vi "ConvertTextBasedCodeToLabVIEW.vi"() -> ()   [LabVIEW 2012]
uses:
  <resource>/Framework/Providers/Open_GDS/ClassProviders/Common/String/GDSString_ClassDescriptionType.ctl
  <resource>/Framework/Providers/Open_GDS/ClassProviders/Common/String/GDSString_AccessScopeModifierType.ctl
  <resource>/Framework/Providers/Open_GDS/ClassProviders/Common/String/GDSString_ModifierType.ctl
  <resource>/Framework/Providers/Open_GDS/ClassProviders/Common/String/GDSString_MethodDescriptionType.ctl
  <resource>/Framework/Providers/Open_GDS/ClassProviders/Common/String/GDSString_ClassParentType.ctl
  <resource>/Framework/Providers/Open_GDS/ClassProviders/Common/String/GDSString_ClassType.ctl
  <resource>/Framework/Providers/Open_GDS/ClassProviders/Common/String/GDSString_ClassOwnerType.ctl
  <resource>/Framework/Providers/Open_GDS/ClassProviders/Common/CommonVIs/CommonVIs_AttributeType.ctl
  <resource>/Framework/Providers/Open_GDS/ClassProviders/Common/CommonVIs/CommonVIs_AttributeDataType.ctl
  <resource>/Framework/Providers/Open_GDS/ClassProviders/Common/CommonVIs/CommonVIs_EnumType.ctl
  <resource>/Framework/Providers/Open_GDS/ClassProviders/Common/CommonVIs/CommonVIs_StructType.ctl
  <vilib>/Utility/miscctls.llb/LVPointTypeDef.ctl
  <vilib>/Platform/browser.llb/Open URL in Default Browser (path).vi
panel:
  out "Array":T1[](array[typedef])
  out "Classes":T4[](array[typedef])
  out "Tab":T12(tab)
  in  "RemoveSelectedFiles":bool
  in  "ClearList":bool
  in  "FileList":i32[](listbox) caption="File List"
  in  "CopyfromClipboard":bool
  in  "Code":string caption="Java or C# Code"
  in  "Path":path caption="Java or C# File or top level folder"
  out "FileListText":bool
  in  "Missing":i32(listbox) caption="Missing Classes and types"
  in  "ViewClassOverView":bool
  in  "ClassType":T13(ring) caption="Class Type"
  in  "TopFolder":path caption="Top Folder for all classes"
  in  "Previous":bool
  in  "Cancel":bool
  in  "Next":bool
  out "error IO":errorcluster
  # "There are some missing classes/types that could not be found.\nDo you want to contine?\nYou can go back and add some more files that might contain the missing types."
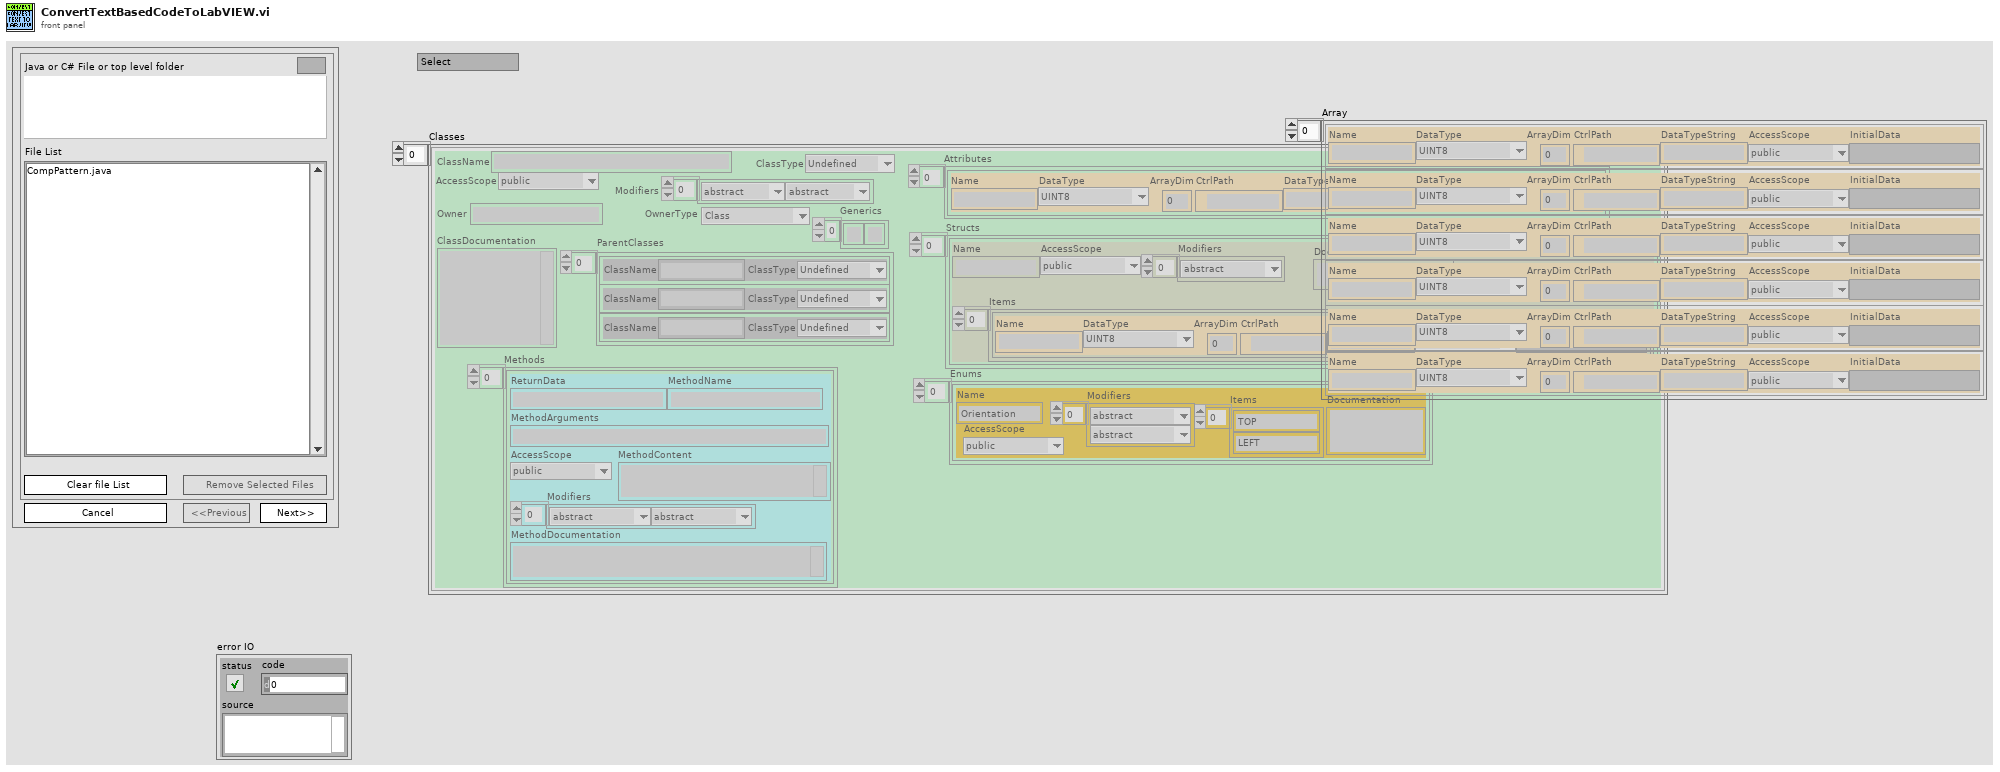
[diagram p1: front panel]
types:
  T1 = typedef "CommonVIs_AttributeType.ctl" = cluster{"Name":string, "DataType":T2, "ArrayDim":i32, "CtrlPath":path, "DataTypeString":string, "AccessScope":T3, "InitialData":variant}
  T2 = typedef "CommonVIs_AttributeDataType.ctl" = enum16{"UINT8", "INT8", "UINT16", "INT16", "UINT32", "INT32", "UINT64", "INT64", "SGL", "DBL", "EXT", "CSG", "CDB", "CXT", "TimeStamp", "STRING", "PATH", "BOOL", "ENUM", "RefNum", "VIRefNum", "LabVIEW Class", "Cluster", "Variant", "TypeDef", "Waveform", "LabVIEW Object", "Other"}
  T3 = typedef "GDSString_AccessScopeModifierType.ctl" = enum16{"public", "private", "protected", "internal"}
  T4 = typedef "GDSString_ClassDescriptionType.ctl" = cluster{"ClassName":string, "AccessScope":T3, "Modifiers":T5[], "ClassDocumentation":string, "Methods":T6[], "ParentClasses":T7[], "ClassType":T8, "Owner":string, "OwnerType":T9, "Generics":string[], "Attributes":T1[], "Enums":T10[], "Structs":T11[]}
  T5 = typedef "GDSString_ModifierType.ctl" = enum16{"abstract", "static", "final", "synchronized", "strictfp", "async", "const", "event", "extern", "new", "override", "partial", "readonly", "sealed", "unsafe", "virtual", "volatile"}
  T6 = typedef "GDSString_MethodDescriptionType.ctl" = cluster{"ReturnData":string, "MethodName":string, "MethodArguments":string, "AccessScope":T3, "Modifiers":T5[], "MethodDocumentation":string, "MethodContent":string}
  T7 = typedef "GDSString_ClassParentType.ctl" = cluster{"ClassName":string, "ClassType":T8}
  T8 = typedef "GDSString_ClassType.ctl" = enum16{"Undefined", "Class", "Interface"}
  T9 = typedef "GDSString_ClassOwnerType.ctl" = enum16{"NoOwner", "Class", "Package/NameSpace"}
  T10 = typedef "CommonVIs_EnumType.ctl" = cluster{"Name":string, "AccessScope":T3, "Modifiers":T5[], "Items":string[], "Documentation":string}
  T11 = typedef "CommonVIs_StructType.ctl" = cluster{"Name":string, "AccessScope":T3, "Modifiers":T5[], "Items":T1[], "Documentation":string}
  T12 = enum32{"Select", "Analysing", "Missing", "Overview"}
  T13 = enum16{"Native By Value LabVIEW Classes", "Reference Object DVR (GOOP4)", "Reference Object  (GOOP3)"}
  T14 = typedef "LVPointTypeDef.ctl" = cluster{"Horizontal":i16, "Vertical":i16}
  T15 = cluster{"Counter":i32, "Text":string, "Cancelled":bool, "Files":path[], "Classes":T4[]}
  T16 = enum8{"Enabled", "Disabled", "Disabled and Grayed Out"}
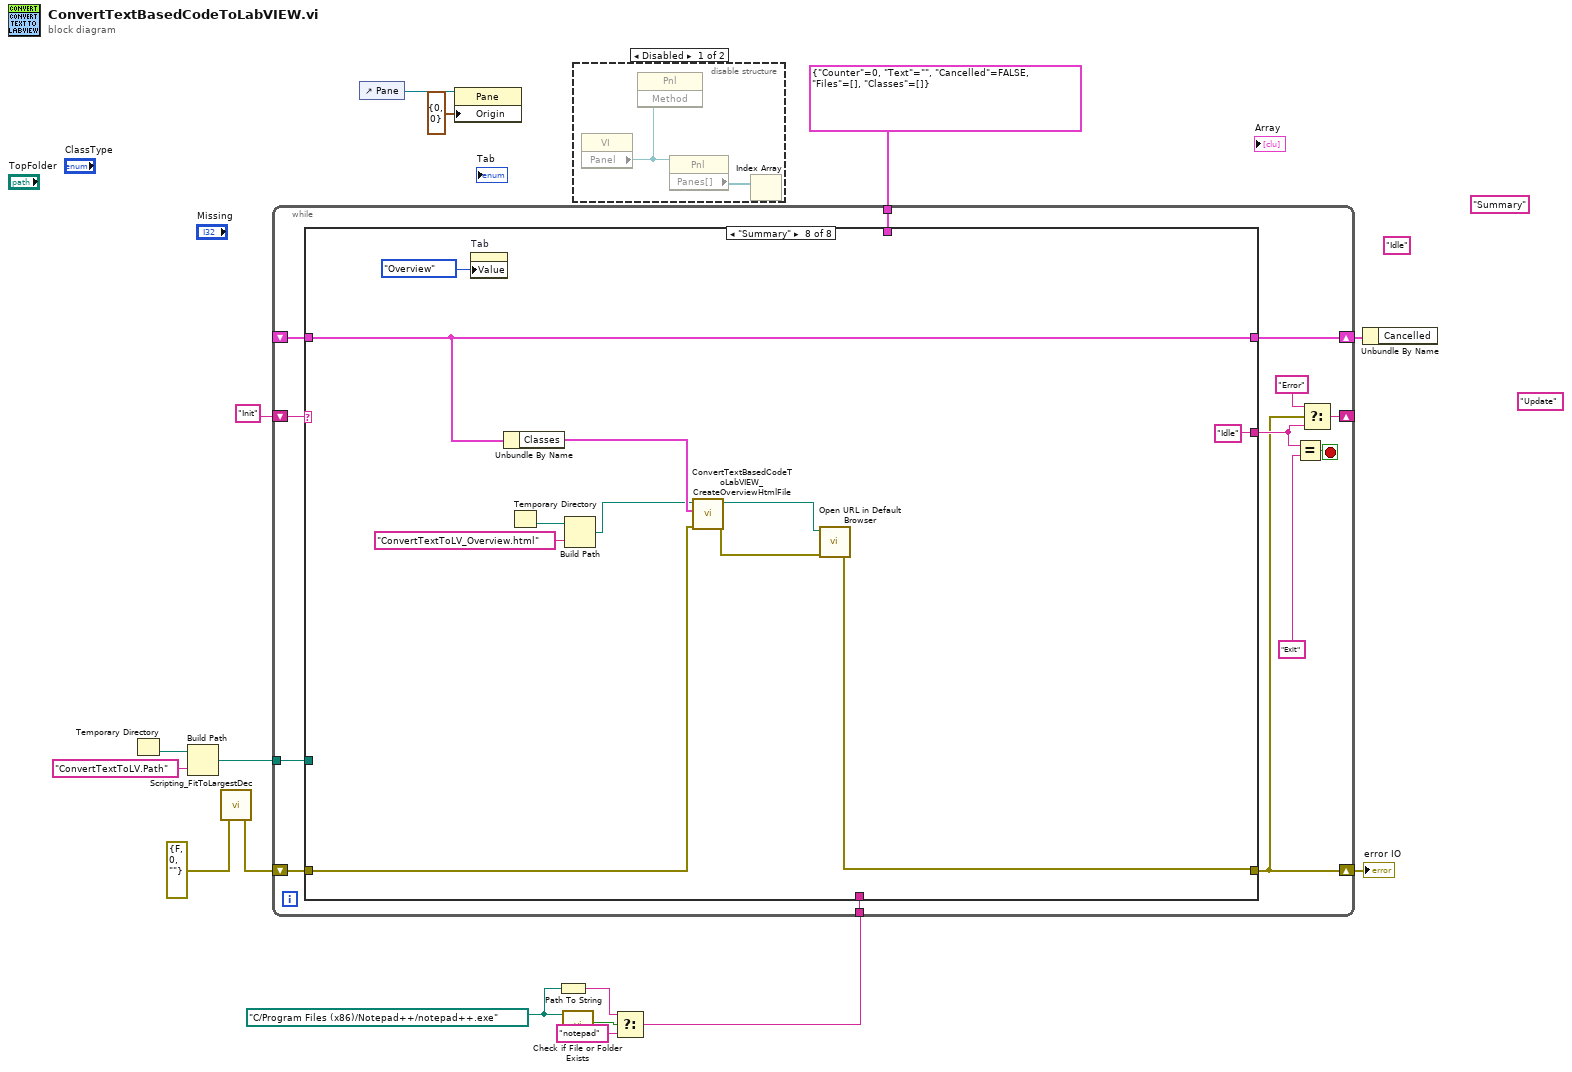
[diagram p0: block diagram]
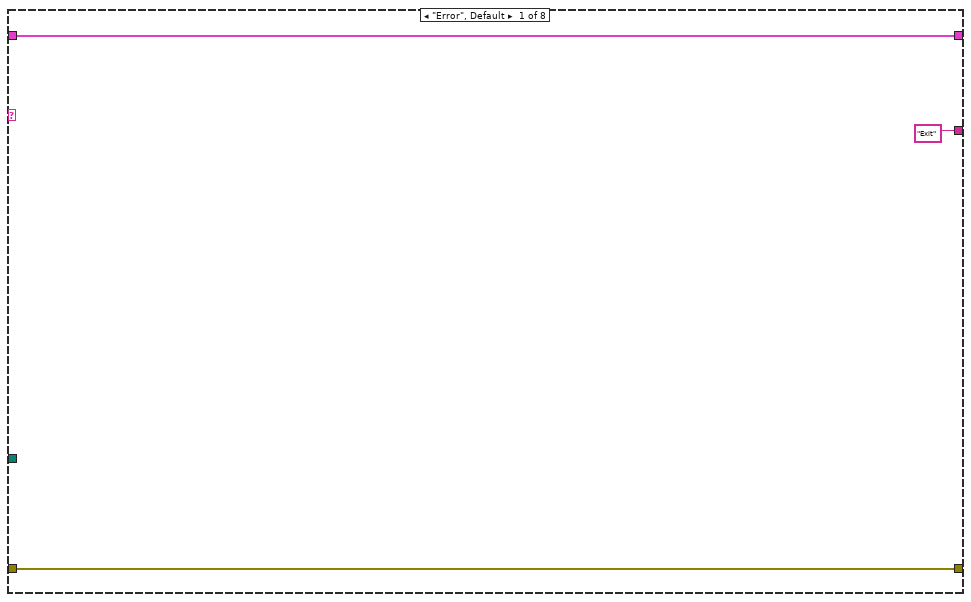
[diagram p3: hidden frame]
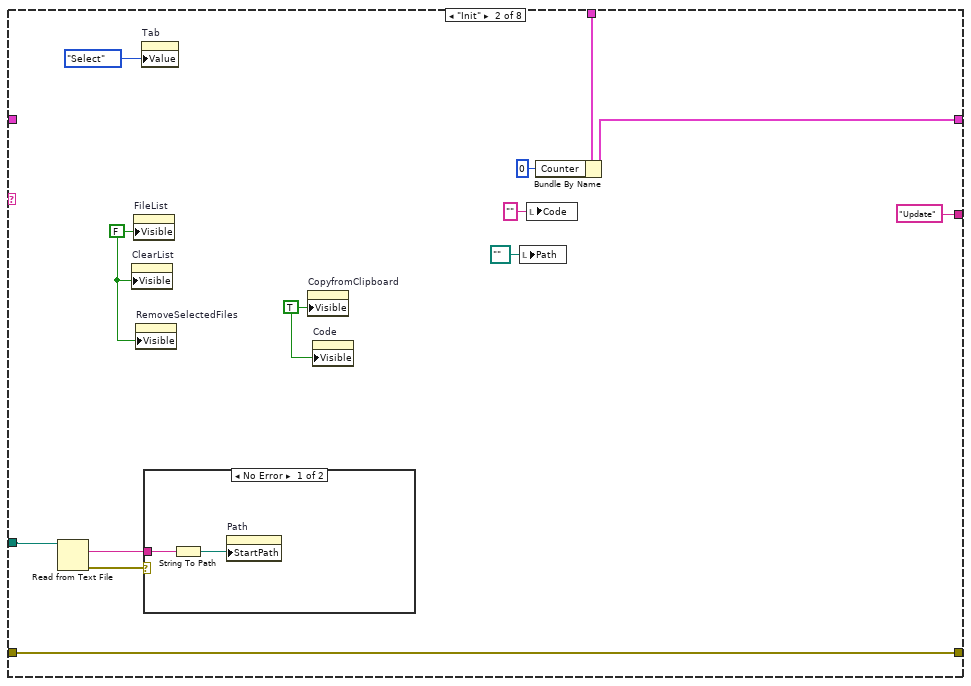
[diagram p4: hidden frame]
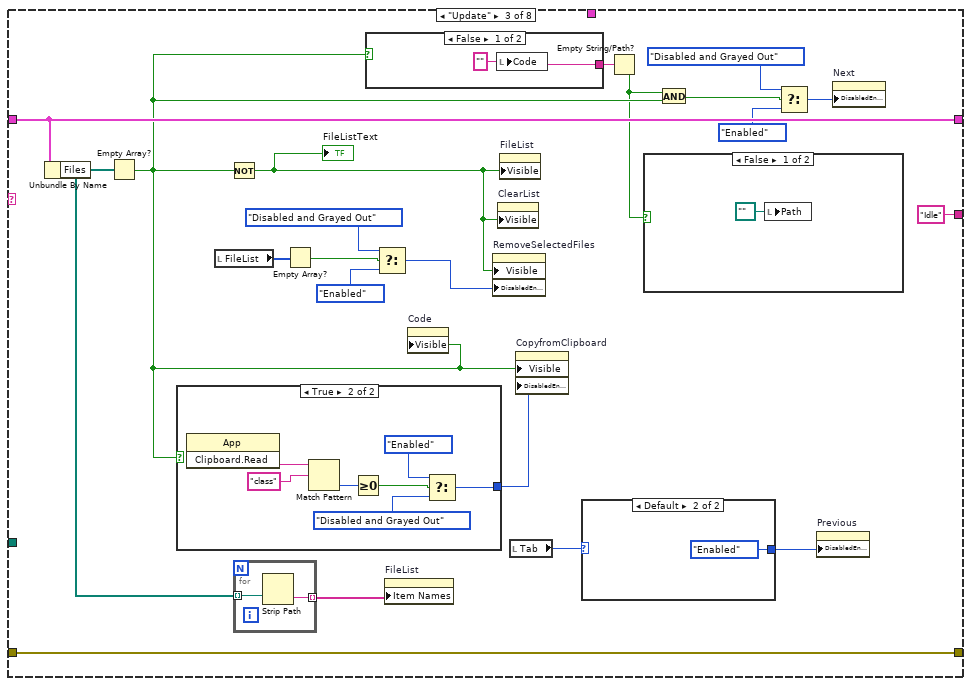
[diagram p6: hidden frame]
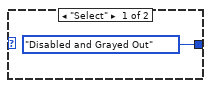
[diagram p7: hidden frame]
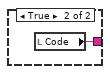
[diagram p9: hidden frame]
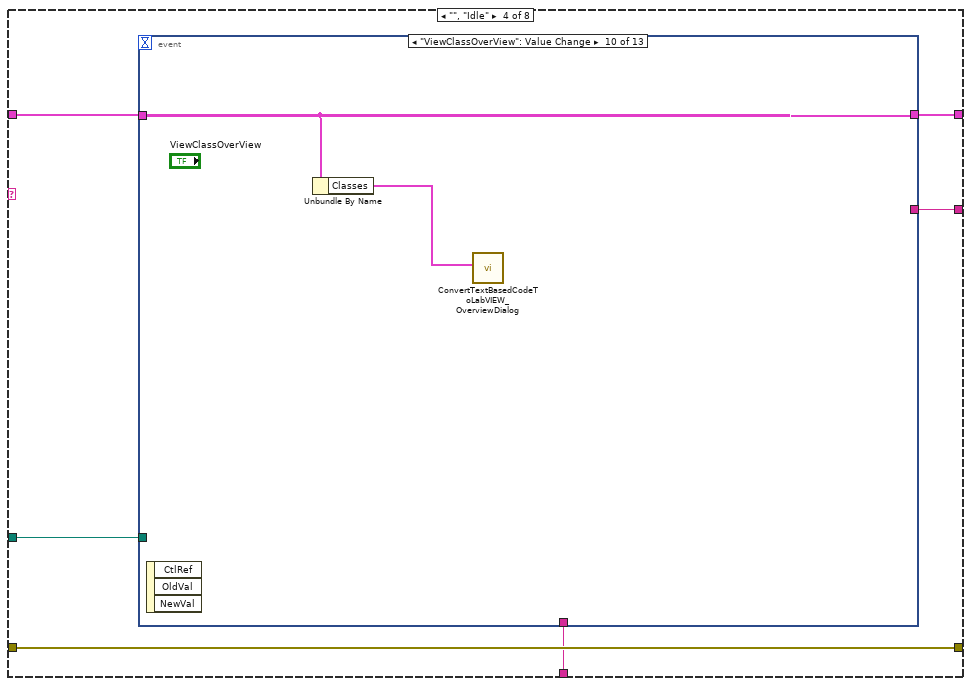
[diagram p11: hidden frame]
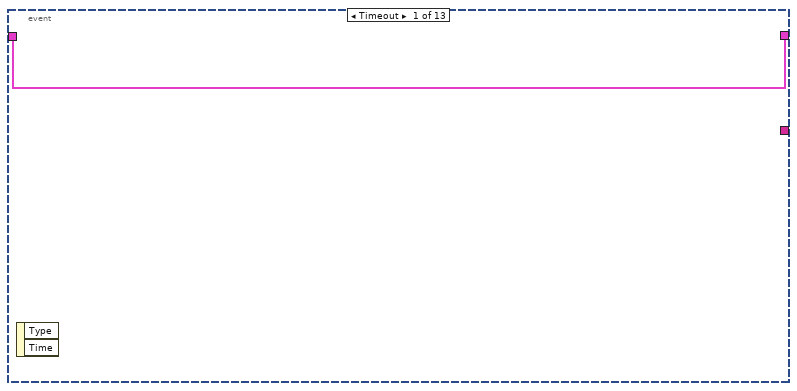
[diagram p12: hidden frame]
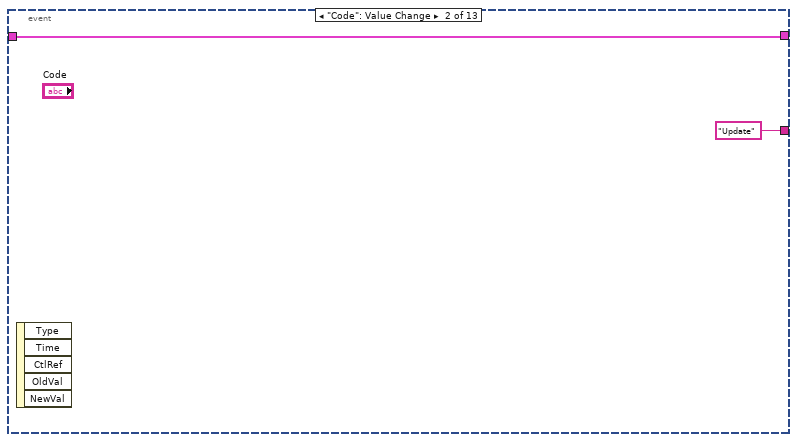
[diagram p13: hidden frame]
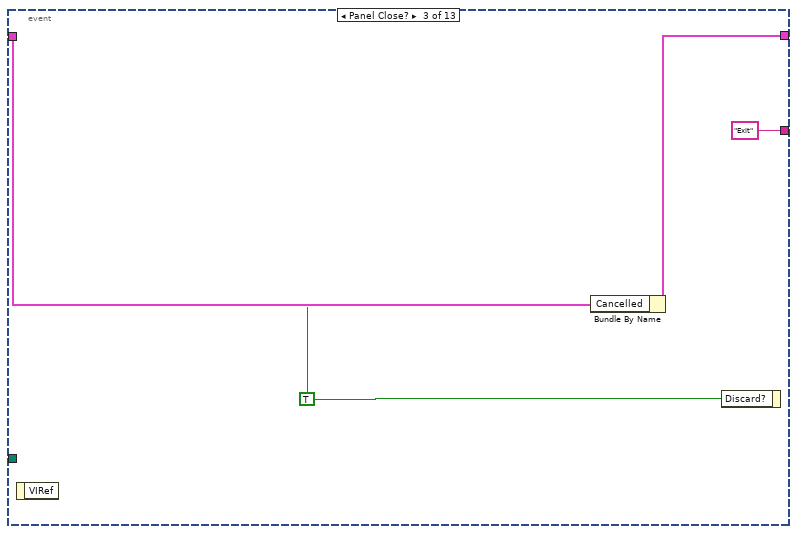
[diagram p14: hidden frame]
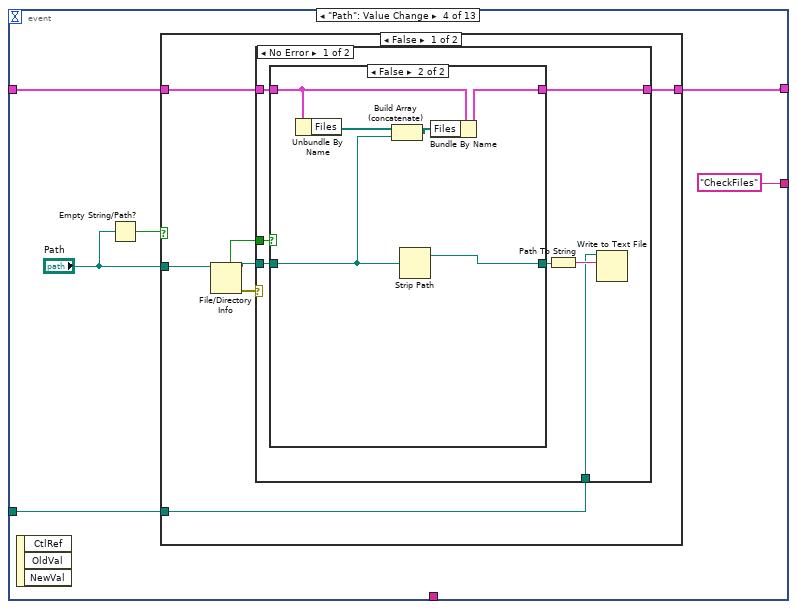
[diagram p15: hidden frame]
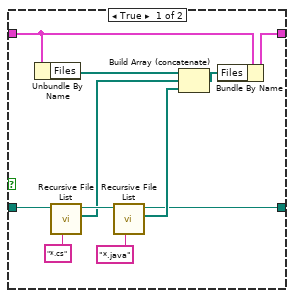
[diagram p16: hidden frame]
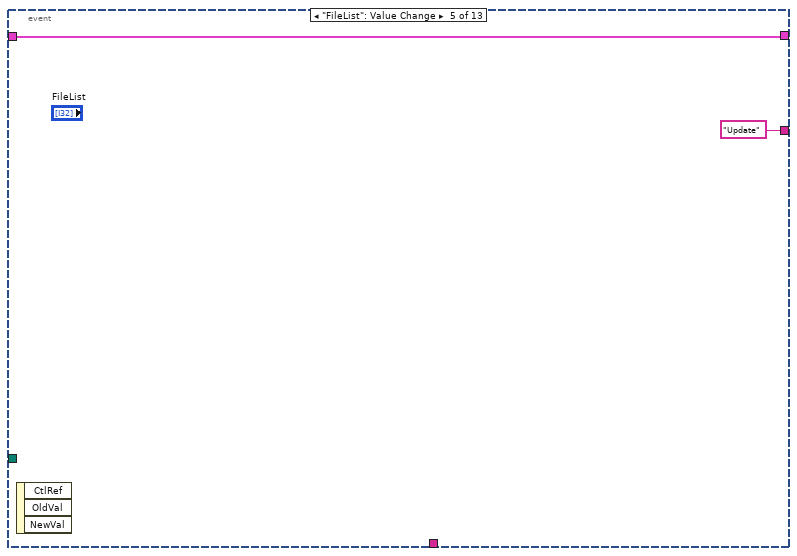
[diagram p19: hidden frame]
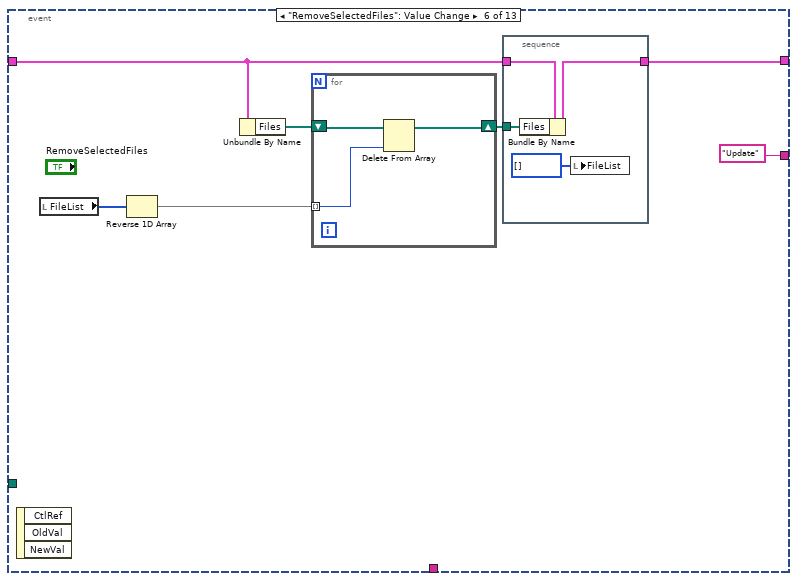
[diagram p20: hidden frame]
diagram:
  w4 = path "C:/Program Files (x86)/Notepad++/notepad++.exe"
  (unwired) "Update"
  (unwired) "Idle"
  (unwired) "Summary"
  n1 = Temporary Directory() -> (w9:path)
  n2 = Build Path(base path=w9, name or relative path="ConvertTextToLV.Path") -> (appended path=w8:path)
  n3 = call <resource>:"Scripting_FitToLargestDec.vi"("error in (no error)"=errorcluster {"status"=FALSE, "code"=0, "source"=""} ("error IO")) -> ("error out"=w6:errorcluster)  [unwired: 5 in, 1 out]
  n4 = control-ref of="Pane"() -> (w11:refnum<vi>)
  n5 = property class="Pane"(reference=w11, "Origin"=T14 {"Horizontal"=0, "Vertical"=0}) -> ()  [unwired: 1 in, 2 out]
  n6 = Path To String(path=w4) -> (string=w3:string)
  n7 = call <vilib>:"Check if File or Folder Exists.vi"("path"=w4) -> ("file or folder exists?"=w5:bool)  [unwired: 8 in, 2 out]
  n8 = disable-structure shown="Disabled" {
    frame Disabled {
      n9 = property class="VI"() -> ("Panel"=w18:refnum<vi>)  [unwired: 2 in, 2 out]
      n10 = invoke class="Pnl" method=#-1(reference=w18) -> ()  [unwired: 2 in, 3 out]
      n11 = property class="Pnl"(reference=w18) -> ("Panes[]"=w17:refnum<vi>[])  [unwired: 1 in, 2 out]
      n12 = Index Array(array=w17) -> ()  [unwired: 1 in, 1 out]
    }
    frame Enabled {
    }
  }
  n13 = Select(t=w3, s=w5, f="notepad") -> (s? t:f=w1:string)
  n14 = while {
    shift-right: [w24] -> w14
    shift-left: w6 -> [w31]
    shift-right: [w29] -> _
    shift-left: "Init" -> [w30]
    shift-right: [w23] -> w15
    shift-left: _ -> [w22]
    tunnel: T15 {"Counter"=0, "Text"="", "Cancelled"=FALSE, "Files"=[], "Classes"=[]} -> [w21]
    tunnel: w8 -> [w20]
    tunnel: w1 -> [w19]
    stop <- w28 stop-if-true
    n15 = case shown="\"Summary\"" w30 {
      tunnel: w31 -> [w34 w46 w68 w87 w215 w235 w307 w323]
      tunnel: [w34 w46 w68 w87 w214 w236 w307 w322] -> w24
      tunnel: ["Exit" "Update" "Idle" w88 w207 w237 "Update" "Idle"] -> w25
      tunnel: [w32 w45 w69 w89 w208 w246 w308 w328] -> w23
      tunnel: w22 -> [w32 _ w69 w90 w213 w246 w310 w328]
      tunnel: w21 -> [_ w43 _ _ _ _ _ _]
      tunnel: w20 -> [_ w38 _ w86 _ _ _ _]
      tunnel: w19 -> [_ _ _ w85 _ _ _ _]
      frame "Error", Default {
      }
      frame "Init" {
        w39 = TRUE ("Visible")
        w40 = FALSE ("Visible")
        n16 = Read from Text File(file (use dialog)=w38) -> (text=w36:string, error out=w37:errorcluster)  [unwired: 3 in, 2 out]
        n17 = property on="ClearList" class="Bool"("Visible"=w40) -> ()  [unwired: 2 in, 2 out]
        n18 = property on="FileList" class="LstBox (strict)"("Visible"=w40) -> ()  [unwired: 2 in, 2 out]
        n19 = property on="RemoveSelectedFiles" class="Bool"("Visible"=w40) -> ()  [unwired: 2 in, 2 out]
        n20 = property on="Tab" class="TabCtl (strict)"("Value"=T12."Select" ("Tab")) -> ()  [unwired: 2 in, 2 out]
        n21 = case shown="No Error" w37 {
          tunnel: w36 -> [w49 _]
          frame No Error {
            n22 = String To Path(string=w49) -> (path=w48:path)
            n23 = property on="Path" class="Path"("StartPath"=w48) -> ()  [unwired: 2 in, 2 out]
          }
          frame Error {
          }
        }
        n24 = property on="CopyfromClipboard" class="Bool"("Visible"=w39) -> ()  [unwired: 2 in, 2 out]
        n25 = property on="Code" class="Str"("Visible"=w39) -> ()  [unwired: 2 in, 2 out]
        n26 = local write "Path"(path "" ("Path")) -> ()
        n27 = local write "Code"("" ("Code")) -> ()
        n28 = Bundle By Name(cluster=w43, "Counter"=0) -> (w45:T15)
      }
      frame "Update" {
        n29 = Unbundle By Name(w69) -> ("Files"=w61:path[])
        n30 = Empty Array?(array=w61) -> (empty?=w54:bool)
        n31 = case shown="True" w54 {
          tunnel: [_ w79] -> w67
          frame False {
          }
          frame True {
            n32 = invoke class="App" method="Clipboard.Read"() -> ("Read Clipbrd"=w84:string)  [unwired: 3 in, 2 out]
            n33 = Match Pattern(string=w84, regular expression="class") -> (offset past match=w82:i32)  [unwired: 1 in, 3 out]
            n34 = Greater Or Equal To 0?(x=w82) -> (x >= 0?=w81:bool)
            n35 = Select(t=T16."Enabled" ("Disabled"), s=w81, f=T16."Disabled and Grayed Out" ("Disabled")) -> (s? t:f=w79:T16)
          }
        }
        n36 = local read "FileList"() -> (w66:i32[])
        n37 = Not(x=w54) -> (.not. x?=w50:bool)
        "FileListText" <- w50
        n38 = for {
          tunnel: w61 -> [w77] mode=indexing
          tunnel: [w76] -> w60 mode=indexing
          n39 = Strip Path(path=w77) -> (name=w76:string)  [unwired: 1 out]
        }
        n40 = Empty Array?(array=w66) -> (empty?=w64:bool)
        n41 = case shown="False" w54 {
          tunnel: [w74 w75] -> w59
          frame False {
            w74 = "" ("Code")
            n42 = local write "Code"(w74) -> ()
          }
          frame True {
            n43 = local read "Code"() -> (w75:string)
          }
        }
        n44 = Select(t=T16."Disabled and Grayed Out" ("Disabled"), s=w64, f=T16."Enabled" ("Disabled")) -> (s? t:f=w62:T16)
        n45 = property on="FileList" class="LstBox (strict)"("Item Names"=w60) -> ()  [unwired: 2 in, 2 out]
        n46 = property on="Code" class="Str"("Visible"=w54) -> ()  [unwired: 2 in, 2 out]
        n47 = property on="RemoveSelectedFiles" class="Bool"("Visible"=w50, "DisabledEnum"=w62) -> ()  [unwired: 2 in, 2 out]
        n48 = property on="ClearList" class="Bool"("Visible"=w50) -> ()  [unwired: 2 in, 2 out]
        n49 = property on="FileList" class="LstBox (strict)"("Visible"=w50) -> ()  [unwired: 2 in, 2 out]
        n50 = local read "Tab"() -> (w52:T12)
        n51 = property on="CopyfromClipboard" class="Bool"("Visible"=w54, "DisabledEnum"=w67) -> ()  [unwired: 2 in, 2 out]
        n52 = case shown="Default" w52 {
          tunnel: [T16."Disabled and Grayed Out" ("Disabled") T16."Enabled" ("Disabled")] -> w51
          frame "Select" {
          }
          frame Default {
          }
        }
        n53 = Empty String/Path?(string/path=w59) -> (empty?=w53:bool)
        n54 = case shown="False" w53 {
          frame False {
            n55 = local write "Path"(path "" ("Path")) -> ()
          }
          frame True {
          }
        }
        n56 = And(x=w53, y=w54) -> (x .and. y?=w56:bool)
        n57 = Select(t=T16."Disabled and Grayed Out" ("Disabled"), s=w56, f=T16."Enabled" ("Disabled")) -> (s? t:f=w55:T16)
        n58 = property on="Previous" class="Bool"("DisabledEnum"=w51) -> ()  [unwired: 2 in, 2 out]
        n59 = property on="Next" class="Bool"("DisabledEnum"=w55) -> ()  [unwired: 2 in, 2 out]
      }
      frame "", "Idle" {
        n60 = event shown="[9] \"ViewClassOverView\": Value Change" {
          selector: _ -> [_ _ _ _ _ _ _ _ _ _ _ _ _]
          dyn-events: _ -> [_ _ _ _ _ _ _ _ _ _ _ _ _]
          timeout: _ -> [_ _ _ _ _ _ _ _ _ _ _ _ _]
          tunnel: w90 -> [w91 w93 w96 w101 w138 w144 w157 w178 w181 w187 w190 w196 w201]
          tunnel: [w91 w93 w95 w100 w138 w145 w158 w178 w181 w187 w190 w196 w202] -> w89
          tunnel: [_ "Update" "Exit" "CheckFiles" "Update" "Update" "Update" "Update" w180 _ w189 "Exit" "Update"] -> w88
          tunnel: w86 -> [_ _ _ w98 _ _ _ _ _ _ _ _ _]
          tunnel: w85 -> [_ _ _ _ _ _ w153 _ _ _ _ _ _]
          event Timeout {
            n61 = event-data() -> ()  [unwired: 1 in, 2 out]
          }
          event "Code": Value Change {
            n62 = event-data() -> ()  [unwired: 1 in, 5 out]
          }
          event Panel Close? {
            w94 = TRUE ("Discard?")
            n63 = event-data() -> ()  [unwired: 1 in, 1 out]
            n64 = Bundle By Name(cluster=w96, "Cancelled"=w94) -> (w95:T15)
            n65 = event-data("Discard?"=w94) -> ()  [unwired: 1 in, 1 out]
          }
          event "Path": Value Change {
            n66 = event-data() -> ()  [unwired: 1 in, 3 out]
            n67 = Empty String/Path?(string/path="Path") -> (empty?=w102:bool)
            n68 = case shown="False" w102 {
              tunnel: "Path" -> [w110 _]
              tunnel: w101 -> [w108 w136]
              tunnel: [w106 w136] -> w100
              tunnel: w98 -> [w104 _]
              frame False {
                n69 = File/Directory Info(path=w110) -> (path out=w107:path, directory=w109:bool, error out=w105:errorcluster)  [unwired: 1 in, 4 out]
                n70 = case shown="No Error" w105 {
                  tunnel: w109 -> [w117 _]
                  tunnel: w108 -> [w116 w135]
                  tunnel: w107 -> [w115 _]
                  tunnel: [w114 w135] -> w106
                  tunnel: w104 -> [w111 _]
                  frame No Error {
                    n71 = case shown="False" w117 {
                      tunnel: w116 -> [w123 w133]
                      tunnel: w115 -> [w126 w130]
                      tunnel: [w124 w134] -> w114
                      tunnel: [w118 w129] -> w112
                      frame True {
                        n72 = Unbundle By Name(w123) -> ("Files"=w122:path[])
                        n73 = call <vilib>:"Recursive File List.vi"("pattern"="*.cs", "Folder Path"=w126) -> ("All Files in Dir"=w120:path[], "dup Folder Path"=w125:path)  [unwired: 5 in, 3 out]
                        n74 = call <vilib>:"Recursive File List.vi"("pattern"="*.java", "Folder Path"=w125) -> ("All Files in Dir"=w119:path[], "dup Folder Path"=w118:path)  [unwired: 5 in, 3 out]
                        n75 = Build Array (concatenate)(w122, w120, w119) -> (w121:path[])
                        n76 = Bundle By Name(cluster=w123, "Files"=w121) -> (w124:T15)
                      }
                      frame False {
                        n77 = Unbundle By Name(w133) -> ("Files"=w132:path[])
                        n78 = Build Array (concatenate)(w132, w130) -> (w131:path[])
                        n79 = Strip Path(path=w130) -> (stripped path=w129:path)  [unwired: 1 out]
                        n80 = Bundle By Name(cluster=w133, "Files"=w131) -> (w134:T15)
                      }
                    }
                    n81 = Path To String(path=w112) -> (string=w113:string)
                    n82 = Write to Text File(file (use dialog)=w111, text=w113) -> ()  [unwired: 2 in, 3 out]
                  }
                  frame Error {
                  }
                }
              }
              frame True {
              }
            }
          }
          event "FileList": Value Change {
            n83 = event-data() -> ()  [unwired: 1 in, 3 out]
          }
          event "RemoveSelectedFiles": Value Change {
            n84 = event-data() -> ()  [unwired: 1 in, 3 out]
            n85 = local read "FileList"() -> (w142:i32[])
            n86 = Reverse 1D Array(array=w142) -> (reversed array=w140:i32[])
            n87 = Unbundle By Name(w144) -> ("Files"=w143:path[])
            n88 = for {
              shift-right: [w151] -> w141
              shift-left: w143 -> [w152]
              tunnel: w140 -> [w150] mode=indexing
              n89 = Delete From Array(array=w152, index=w150) -> (array with subset deleted=w151:path[])  [unwired: 1 in, 1 out]
            }
            n90 = stacked-sequence {
              tunnel: [w149] -> w145
              tunnel: w144 -> [w148]
              tunnel: w141 -> [w147]
              frame #0 {
                n91 = Bundle By Name(cluster=w148, "Files"=w147) -> (w149:T15)
                n92 = local write "FileList"(i32[] [] ("FileList")) -> ()
              }
            }
          }
          event "FileList": Double Click {
            n93 = event-data() -> ("Row"=w155:i32, "PlatMods.Ctrl"=w154:bool)  [unwired: 1 in]
            n94 = case shown="True" w154 {
              tunnel: [w163 w174] -> w158
              tunnel: w157 -> [w162 w174]
              tunnel: w155 -> [w159 w173]
              tunnel: w153 -> [_ w168]
              frame False {
                n95 = Unbundle By Name(w162) -> ("Files"=w161:path[])
                n96 = Delete From Array(array=w161, index=w159) -> (array with subset deleted=w160:path[])  [unwired: 1 in, 1 out]
                n97 = stacked-sequence {
                  tunnel: [w167] -> w163
                  tunnel: w162 -> [w166]
                  tunnel: w160 -> [w165]
                  frame #0 {
                    n98 = Bundle By Name(cluster=w166, "Files"=w165) -> (w167:T15)
                    n99 = local write "FileList"(i32[] [] ("FileList")) -> ()
                  }
                }
              }
              frame True {
                n100 = Unbundle By Name(w174) -> ("Files"=w175:path[])
                n101 = Index Array(array=w175, index=w173) -> (element=w172:path)
                n102 = Format Into String(format string=" \"%s\"", initial string=w168, w172) -> (resulting string=w169:string)  [unwired: 1 in, 1 out]
                n103 = call <vilib>:"System Exec.vi"("wait until completion? (T)"=TRUE, "command line"=w169) -> ()  [unwired: 6 in, 4 out]
              }
            }
          }
          event "CopyfromClipboard": Value Change {
            n104 = event-data() -> ()  [unwired: 1 in, 3 out]
            n105 = invoke class="App" method="Clipboard.Read"() -> ("Read Clipbrd"=w177:string)  [unwired: 3 in, 2 out]
            n106 = local write "Code"(w177) -> ()
          }
          event "Next": Value Change {
            n107 = event-data() -> ()  [unwired: 1 in, 3 out]
            n108 = local read "Tab"() -> (w179:T12)
            n109 = case shown="\"Overview\"" w179 {
              tunnel: ["AnalyseFiles" "Summary" "Idle" "CreateClasses"] -> w180
              frame "Select" {
              }
              frame "Missing" {
              }
              frame Default {
              }
              frame "Overview" {
              }
            }
          }
          event "ViewClassOverView": Value Change {
            n110 = event-data() -> ()  [unwired: 1 in, 3 out]
            n111 = Unbundle By Name(w187) -> ("Classes"=w186:T4[])
            n112 = call <resource>:"ConvertTextBasedCodeToLabVIEW_OverviewDialog.vi"("ClassesIn"=w186) -> ()  [unwired: 10 in, 1 out]
          }
          event "Previous": Value Change {
            n113 = event-data() -> ()  [unwired: 1 in, 3 out]
            n114 = local read "Tab"() -> (w188:T12)
            n115 = case shown="\"Missing\", \"Overview\"" w188 {
              tunnel: ["AnalyseFiles" "Update" "Idle"] -> w189
              frame "Select" {
              }
              frame "Missing", "Overview" {
                n116 = property on="Tab" class="TabCtl (strict)"("Value"=T12."Select" ("Tab")) -> ()  [unwired: 2 in, 2 out]
              }
              frame Default {
              }
            }
          }
          event "Cancel": Value Change {
            n117 = event-data() -> ()  [unwired: 1 in, 3 out]
          }
          event "ClearList": Value Change {
            n118 = event-data() -> ()  [unwired: 1 in, 3 out]
            n119 = local write "FileList"(i32[] [] ("FileList")) -> ()
            n120 = local write "Path"(path "" ("Path")) -> ()
            n121 = Bundle By Name(cluster=w201, "Files"=path[] []) -> (w202:T15)
          }
        }
      }
      frame "AnalyseFiles" {
        w203 = T12."Analysing" ("Tab")
        n122 = Unbundle By Name(w213) -> ("Files"=w210:path[])
        n123 = local read "Code"() -> (w212:string)
        n124 = call <vilib>:"Trim Whitespace.vi"("string"=w212) -> ("trimmed string"=w211:string)  [unwired: 1 in]
        n125 = call <vilib>:"Set Busy.vi"("error in (no error)"=w215) -> ("error out"=w206:errorcluster)  [unwired: 9 in, 1 out]
        n126 = property on="Tab" class="TabCtl (strict)"("Value"=w203) -> ()  [unwired: 2 in, 2 out]
        n127 = case shown="\"\"" w211 {
          selector: w211 -> [w228 _]
          tunnel: w210 -> [_ w231]
          tunnel: [w226 w231] -> w209
          tunnel: w203 -> [_ _]
          frame Default {
            n128 = Temporary Directory() -> (w229:path)
            n129 = Build Path(base path=w229, name or relative path="GDS_CodeTempFile.txt") -> (appended path=w227:path)
            n130 = Write to Text File(file (use dialog)=w227, text=w228) -> ()  [unwired: 2 in, 3 out]
            n131 = Build Array(w227) -> (w226:path[])
          }
          frame "" {
          }
        }
        n132 = for {
          shift-right: [w225] -> w214
          shift-left: w206 -> [w222]
          tunnel: w209 -> [w223] mode=indexing
          tunnel: [w220] -> w205 mode=concatenating
          n133 = Read from Text File(file (use dialog)=w223, error in=w222) -> (text=w224:string, error out=w221:errorcluster)  [unwired: 2 in, 2 out]
          n134 = call <resource>:"GDSString_ParseTextBasedCode.vi"("error in (no error)"=w221, "TextIn"=w224) -> ("error out"=w225:errorcluster, "Classes"=w220:T4[])  [unwired: 8 in]
        }
        "Classes" <- w205
        n135 = Empty Array?(array=w205) -> (empty?=w204:bool)
        n136 = case shown="False" w204 {
          tunnel: ["CheckDependencies" "Update"] -> w207
          frame False {
          }
          frame True {
            n137 = property on="Tab" class="TabCtl (strict)"("Value"=T12."Select" ("Tab")) -> ()  [unwired: 2 in, 2 out]
            n138 = One Button Dialog(message="No classes found") -> ()  [unwired: 1 in, 1 out]
            n139 = call <vilib>:"Unset Busy.vi"() -> ()  [unwired: 11 in, 1 out]
          }
        }
        n140 = Bundle By Name(cluster=w213, "Classes"=w205) -> (w208:T15)
      }
      frame "CheckDependencies" {
        w243 = T2[] [enum."LabVIEW Class", enum."Other", enum."TypeDef"] items=["UINT8", "INT8", "UINT16", "INT16", "UINT32", "INT32", "UINT64", "INT64", "SGL", "DBL", "EXT", "CSG", "CDB", "CXT", "TimeStamp", "STRING", "PATH", "BOOL", "ENUM", "RefNum", "VIRefNum", "LabVIEW Class", "Cluster", "Variant", "TypeDef", "Waveform", "LabVIEW Object", "Other"] ("1D array")
        n141 = Unbundle By Name(w246) -> ("Classes"=w245:T4[])
        n142 = for {
          tunnel: w245 -> [w281] mode=indexing
          tunnel: [w280] -> w244 mode=indexing
          tunnel: [w277] -> w242 mode=concatenating
          tunnel: w243 -> [w275]
          tunnel: [w272] -> w232 mode=concatenating
          n143 = Unbundle By Name(w281) -> ("Generics"=w272:string[], "ClassName"=w280:string, "ParentClasses"=w279:T7[], "Methods"=w278:T6[])  [unwired: 1 out]
          n144 = for {
            tunnel: w278 -> [w296] mode=indexing
            tunnel: [w288] -> w274 mode=indexing if=w291
            tunnel: [w284] -> w276 mode=concatenating
            tunnel: w275 -> [w289]
            n145 = Unbundle By Name(w296) -> ("ReturnData"=w286:string, "MethodArguments"=w283:string)
            n146 = while {
              shift-right: [w298] -> w285
              shift-left: w286 -> [w304]
              tunnel: [w297] -> _ mode=indexing
              stop <- w301 continue-if-true
              # "Remove Generics"
              n147 = call <resource>:"GDSString_FindCodeBlock.vi"("Text"=w304, "CodeBlockStartCharacter( { )"="<", "CodeBlockEndCharacter( } )"=">") -> ("TextBeforeBlock"=w300:string, "TextAfterBlock"=w299:string, "found"=w301:bool, "BlockText"=w297:string)  [unwired: 8 in, 5 out]
              n148 = Concatenate Strings(w300, w299) -> (w298:string)
            }
            n149 = call <resource>:"GDSString_AttributeTextToAttributeType.vi"("MethodText"=w283, "DefaultAccessScope(Private)"=GDSString_AccessScopeModifierType."public") -> ("ClassesOrTypesDependency"=w284:string[])  [unwired: 6 in, 3 out]
            n150 = call <resource>:"ReversedEngineering_GetDatatypeFromString.vi"("String"=w285) -> ("AttributeDataType"=w292:T2, "DataTypeAsString(Array,default values removed)"=w288:string)  [unwired: 10 in, 3 out]
            n151 = Not Equal?(x="void", y=w285) -> (x != y?=w294:bool)
            n152 = Search 1D Array(1D array=w289, element=w292) -> (index of element=w293:i32)  [unwired: 1 in]
            n153 = Empty String/Path?(string/path=w288) -> (empty?=w287:bool)
            n154 = Greater Or Equal To 0?(x=w293) -> (x >= 0?=w290:bool)
            n155 = Compound Arithmetic op=AND(w294, w290, invert w287) -> (w291:bool)
          }
          n156 = call <resource>:"GDSString_AttributeTextToAttributeType.vi"("DefaultAccessScope(Private)"=GDSString_AccessScopeModifierType."private") -> ("ClassesOrTypesDependency"=w271:string[])  [unwired: 7 in, 3 out]
          n157 = for {
            tunnel: w279 -> [w306] mode=indexing
            tunnel: [w305] -> w273 mode=indexing
            n158 = Unbundle By Name(w306) -> ("ClassName"=w305:string)
          }
          n159 = Build Array (concatenate)(w273, w274, w276, w271) -> (w277:string[])
        }
        n160 = To Upper Case(1:w244) -> (0:w240:string[])
        n161 = for {
          tunnel: w242 -> [w254] mode=indexing
          shift-right: [w261] -> w239
          shift-left: string[] [] -> [w262]
          tunnel: w240 -> [w258]
          tunnel: w232 -> [w255]
          n162 = To Upper Case(1:w254) -> (0:w259:string)
          n163 = To Upper Case(1:w262) -> (0:w260:string[])
          n164 = Search 1D Array(1D array=w260, element=w259) -> (index of element=w265:i32)  [unwired: 1 in]
          n165 = Search 1D Array(1D array=w255, element=w254) -> (index of element=w253:i32)  [unwired: 1 in]
          n166 = Search 1D Array(1D array=w258, element=w254) -> (index of element=w257:i32)  [unwired: 1 in]
          n167 = Less Than 0?(x=w253) -> (x < 0?=w252:bool)
          n168 = Less Than 0?(x=w257) -> (x < 0?=w256:bool)
          n169 = Less Than 0?(x=w265) -> (x < 0?=w263:bool)
          n170 = Compound Arithmetic op=AND(w252, w256, w263) -> (w264:bool)
          n171 = case shown="True" w264 {
            tunnel: w262 -> [w266 w269]
            tunnel: w254 -> [_ w268]
            tunnel: [w266 w267] -> w261
            frame False {
            }
            frame True {
              n172 = Build Array (concatenate)(w269, w268) -> (w267:string[])
            }
          }
        }
        n173 = Empty Array?(array=w239) -> (empty?=w238:bool)
        n174 = case shown="False" w238 {
          tunnel: ["Idle" "Summary"] -> w237
          frame False {
            n175 = property on="Previous" class="Bool"("DisabledEnum"=T16."Enabled" ("Disabled")) -> ()  [unwired: 2 in, 2 out]
            n176 = property on="Tab" class="TabCtl (strict)"("Value"=T12."Missing" ("Tab")) -> ()  [unwired: 2 in, 2 out]
          }
          frame True {
            n177 = property on="Tab" class="TabCtl (strict)"("Value"=T12."Overview" ("Tab")) -> ()  [unwired: 2 in, 2 out]
          }
        }
        n178 = property on="Missing" class="LstBox (strict)"(error in=w235, "Item Names"=w239, "Value"=-1 ("Missing")) -> (error out=w234:errorcluster)  [unwired: 1 in, 1 out]
        n179 = call <vilib>:"Unset Busy.vi"("error in (no error)"=w234) -> ("error out"=w236:errorcluster)  [unwired: 10 in]
      }
      frame "CheckFiles" {
        n180 = Unbundle By Name(w310) -> ("Files"=w312:path[])
        n181 = for {
          tunnel: w312 -> [w315] mode=indexing
          shift-right: [w314] -> w309
          shift-left: path[] [] -> [w316]
          n182 = Search 1D Array(1D array=w316, element=w315) -> (index of element=w317:i32)  [unwired: 1 in]
          n183 = case shown="0, Default" w317 {
            tunnel: w316 -> [w318 w321]
            tunnel: w315 -> [_ w320]
            tunnel: [w318 w319] -> w314
            frame 0, Default {
            }
            frame -1 {
              n184 = Build Array (concatenate)(w321, w320) -> (w319:path[])
            }
          }
        }
        n185 = Bundle By Name(cluster=w310, "Files"=w309) -> (w308:T15)
      }
      frame "Summary" {
        n186 = property on="Tab" class="TabCtl (strict)"("Value"=T12."Overview" ("Tab")) -> ()  [unwired: 2 in, 2 out]
        n187 = Unbundle By Name(w328) -> ("Classes"=w327:T4[])
        n188 = Temporary Directory() -> (w330:path)
        n189 = Build Path(base path=w330, name or relative path="ConvertTextToLV_Overview.html") -> (appended path=w326:path)
        n190 = call <resource>:"ConvertTextBasedCodeToLabVIEW_CreateOverviewHtmlFile.vi"("error in (no error)"=w323, "Classes"=w327, "appended path in"=w326) -> ("error out"=w324:errorcluster, "appended path out"=w325:path)  [unwired: 7 in]
        n191 = call-poly <vilib>:"Open URL in Default Browser.vi"("error in (no error)"=w324, "path"=w325) -> ("error out"=w322:errorcluster)  [unwired: 4 in, 1 out]
      }
    }
    n192 = Equal?(x=w25, y="Exit") -> (x = y?=w28:bool)
    n193 = Select(t="Error", s=w24, f=w25) -> (s? t:f=w29:string)
  }
  "error IO" <- w14
  n194 = Unbundle By Name(w15) -> ()  [unwired: 1 out]
